vi "Drive Train Loop Speed.vi"() -> (3 "FIFO Timeout":i32)   [LabVIEW 2014]
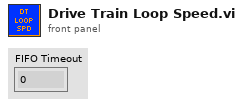
[diagram p1: front panel]
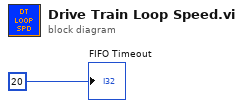
[diagram p0: block diagram]
diagram:
  "FIFO Timeout" <- 20 ("FIFO Timeout")
